vi "Configure Event Search (Serial Bus - USB).vi"(4 "USB PID (0: DATA0/ACK/PING/Out)":i32(ring) items=["DATA0/ACK/PING/Out", "DATA1/NAK/PRE/In", "DATA2/STALL/ERR/Setup", "MDAT/NYET/SPLIT/Sof"], 5 "PID Type (0: Data PID)":i32(ring) items=["Data PID", "Handshake PID", "Special PID", "Token PID"], 6 "Portion of Search Value (XX)":string="XX", 7 "Data Length (4)":dbl=4.0, 8 "error in (no error)":errorcluster, 9 "Portion Target (0: Address)":i32(ring) items=["Address", "CRC", "Data", "4-bit Endpoint", "2-bit ET", "11-bit Frame", "7-bit Hub", "7-bit Port", "1-bit SC", "2-bit S and E or U"], 10 "Search Type (0: Token)":i32(ring) items=["Token", "Data", "Handshake", "Special", "ALL Errors", "PID Error", "CRC5 Error", "CRC16 Error", "Glitch Error", "Stuff Error", "SE1 Error"], 11 "VISA resource name":refnum<visa-resource-name>) -> (0 "error out":errorcluster, 3 "VISA resource name out":refnum<visa-resource-name>)   [LabVIEW 2010, in "Agilent 2000 3000 X-Series.lvlib"]
doc: "Configures the event search of USB bus.\n\n<b>Note(s):</b>\nThis VI is only applicable for Agilent InfiniiVision 4000 X-Series Oscilloscopes."
uses:
  <instrlib>/Agilent 2000 3000 X-Series/Agilent 2000 3000 X-Series.lvlib
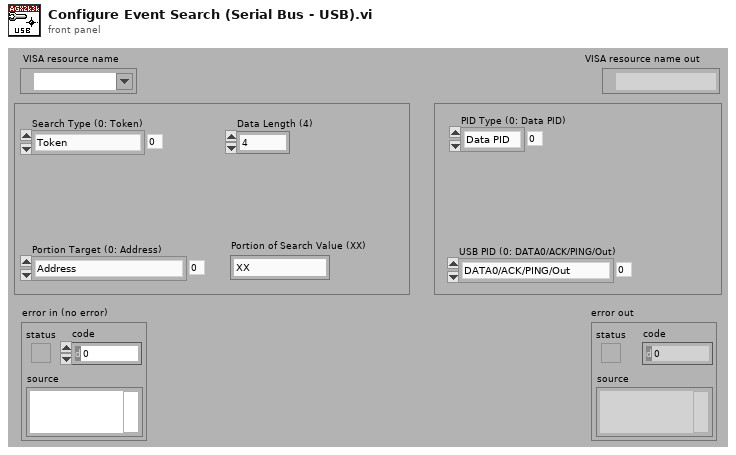
[diagram p1: front panel]
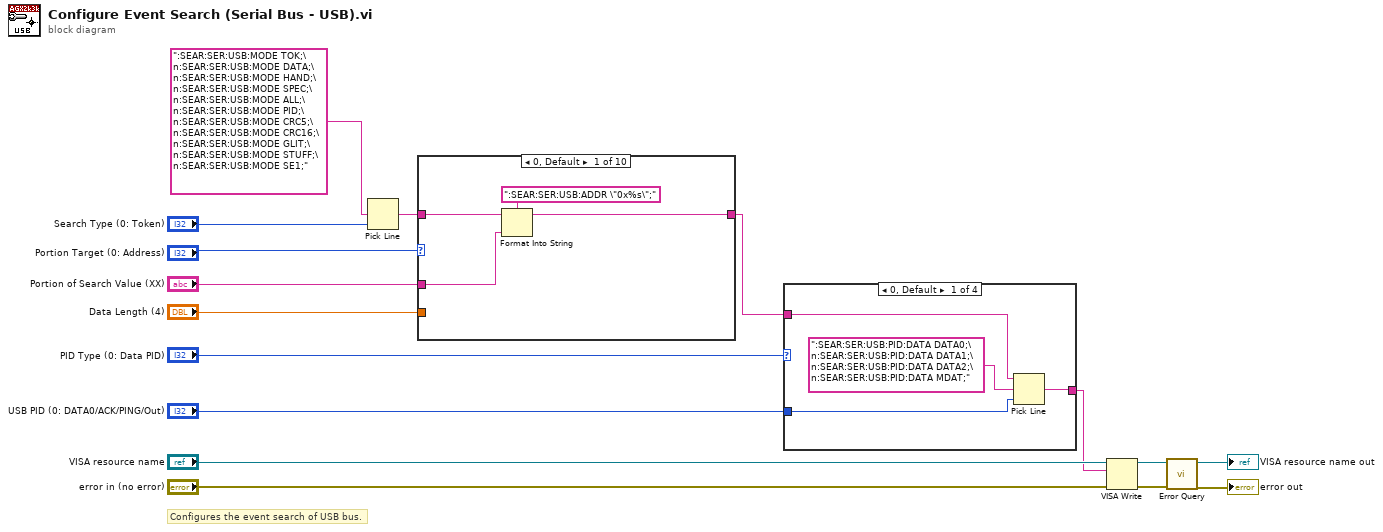
[diagram p0: block diagram]
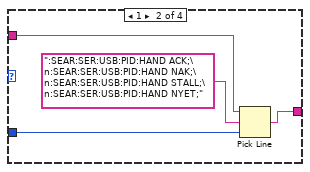
[diagram p2: hidden frame]
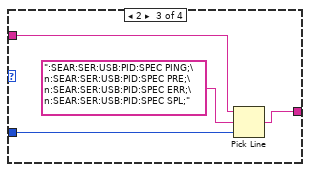
[diagram p3: hidden frame]
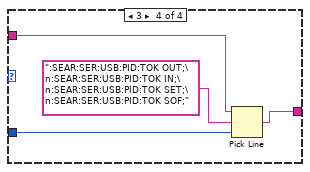
[diagram p4: hidden frame]
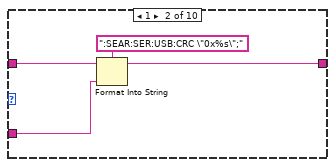
[diagram p5: hidden frame]
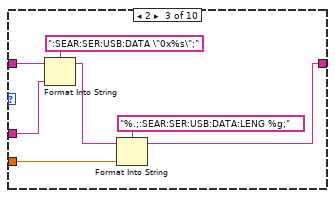
[diagram p6: hidden frame]
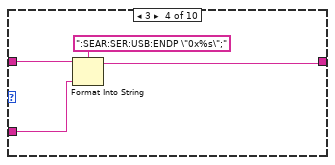
[diagram p7: hidden frame]
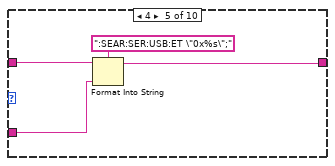
[diagram p8: hidden frame]
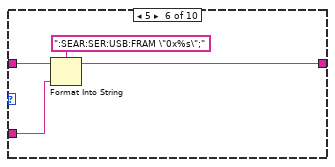
[diagram p9: hidden frame]
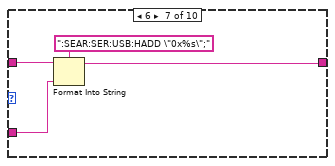
[diagram p10: hidden frame]
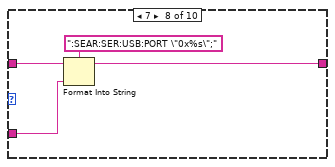
[diagram p11: hidden frame]
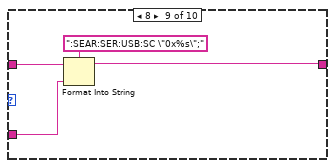
[diagram p12: hidden frame]
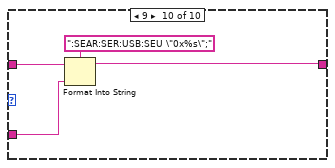
[diagram p13: hidden frame]
diagram:
  # "Configures the event search of USB bus."
  n1 = Pick Line(multi-line string=":SEAR:SER:USB:MODE TOK;\n:SEAR:SER:USB:MODE DATA;\n:SEAR:SER:USB:MODE HAND;\n:SEAR:SER:USB:MODE SPEC;\n:SEAR:SER:USB:MODE ALL;\n:SEAR:SER:USB:MODE PID;\n:SEAR:SER:USB:MODE CRC5;\n:SEAR:SER:USB:MODE CRC16;\n:SEAR:SER:USB:MODE GLIT;\n:SEAR:SER:USB:MODE STUFF;\n:SEAR:SER:USB:MODE SE1;", line index="Search Type (0: Token)") -> (output string=w7:string)  [unwired: 1 out]
  n2 = case shown="0, Default" "Portion Target (0: Address)" {
    tunnel: w7 -> [w19 w23 w30 w34 w38 w42 w46 w50 w54 w58]
    tunnel: [w18 w21 w25 w32 w37 w41 w45 w49 w53 w57] -> w2
    tunnel: "Portion of Search Value (XX)" -> [w17 w22 w29 w33 w36 w40 w44 w48 w52 w56]
    tunnel: "Data Length (4)" -> [_ _ w26 _ _ _ _ _ _ _]
    frame 0, Default {
      n3 = Format Into String(format string=":SEAR:SER:USB:ADDR \"0x%s\";", initial string=w19, w17) -> (resulting string=w18:string)  [unwired: 1 in, 1 out]
    }
    frame 1 {
      n4 = Format Into String(format string=":SEAR:SER:USB:CRC \"0x%s\";", initial string=w23, w22) -> (resulting string=w21:string)  [unwired: 1 in, 1 out]
    }
    frame 2 {
      n5 = Format Into String(format string=":SEAR:SER:USB:DATA \"0x%s\";", initial string=w30, w29) -> (resulting string=w27:string)  [unwired: 1 in, 1 out]
      n6 = Format Into String(format string="%.;:SEAR:SER:USB:DATA:LENG %g;", initial string=w27, w26) -> (resulting string=w25:string)  [unwired: 1 in, 1 out]
    }
    frame 3 {
      n7 = Format Into String(format string=":SEAR:SER:USB:ENDP \"0x%s\";", initial string=w34, w33) -> (resulting string=w32:string)  [unwired: 1 in, 1 out]
    }
    frame 4 {
      n8 = Format Into String(format string=":SEAR:SER:USB:ET \"0x%s\";", initial string=w38, w36) -> (resulting string=w37:string)  [unwired: 1 in, 1 out]
    }
    frame 5 {
      n9 = Format Into String(format string=":SEAR:SER:USB:FRAM \"0x%s\";", initial string=w42, w40) -> (resulting string=w41:string)  [unwired: 1 in, 1 out]
    }
    frame 6 {
      n10 = Format Into String(format string=":SEAR:SER:USB:HADD \"0x%s\";", initial string=w46, w44) -> (resulting string=w45:string)  [unwired: 1 in, 1 out]
    }
    frame 7 {
      n11 = Format Into String(format string=":SEAR:SER:USB:PORT \"0x%s\";", initial string=w50, w48) -> (resulting string=w49:string)  [unwired: 1 in, 1 out]
    }
    frame 8 {
      n12 = Format Into String(format string=":SEAR:SER:USB:SC \"0x%s\";", initial string=w54, w52) -> (resulting string=w53:string)  [unwired: 1 in, 1 out]
    }
    frame 9 {
      n13 = Format Into String(format string=":SEAR:SER:USB:SEU \"0x%s\";", initial string=w58, w56) -> (resulting string=w57:string)  [unwired: 1 in, 1 out]
    }
  }
  n14 = case shown="0, Default" "PID Type (0: Data PID)" {
    tunnel: "USB PID (0: DATA0/ACK/PING/Out)" -> [w62 w66 w70 w74]
    tunnel: w2 -> [w61 w65 w69 w73]
    tunnel: [w60 w64 w68 w72] -> w1
    frame 0, Default {
      n15 = Pick Line(string ("")=w61, multi-line string=":SEAR:SER:USB:PID:DATA DATA0;\n:SEAR:SER:USB:PID:DATA DATA1;\n:SEAR:SER:USB:PID:DATA DATA2;\n:SEAR:SER:USB:PID:DATA MDAT;", line index=w62) -> (output string=w60:string)
    }
    frame 1 {
      n16 = Pick Line(string ("")=w65, multi-line string=":SEAR:SER:USB:PID:HAND ACK;\n:SEAR:SER:USB:PID:HAND NAK;\n:SEAR:SER:USB:PID:HAND STALL;\n:SEAR:SER:USB:PID:HAND NYET;", line index=w66) -> (output string=w64:string)
    }
    frame 2 {
      n17 = Pick Line(string ("")=w69, multi-line string=":SEAR:SER:USB:PID:SPEC PING;\n:SEAR:SER:USB:PID:SPEC PRE;\n:SEAR:SER:USB:PID:SPEC ERR;\n:SEAR:SER:USB:PID:SPEC SPL;", line index=w70) -> (output string=w68:string)
    }
    frame 3 {
      n18 = Pick Line(string ("")=w73, multi-line string=":SEAR:SER:USB:PID:TOK OUT;\n:SEAR:SER:USB:PID:TOK IN;\n:SEAR:SER:USB:PID:TOK SET;\n:SEAR:SER:USB:PID:TOK SOF;", line index=w74) -> (output string=w72:string)
    }
  }
  n19 = VISA Write(VISA resource name="VISA resource name", write buffer=w1, error in (no error)="error in (no error)") -> (VISA resource name out=w12:refnum<visa-resource-name>, error out=w11:errorcluster)  [unwired: 1 out]
  n20 = call <instrlib>:"Error Query.vi"("error in (no error)"=w11, "VISA resource name"=w12) -> ("error out"=→"error out":errorcluster, "VISA resource name out"=→"VISA resource name out":refnum<visa-resource-name>)  [unwired: 8 out]
